vi "element_editor_hydrolysis_initial.vi"(9 "Env. Dir":refnum<vi>, 10 "Env. Ready?":refnum<vi>, 11 "Break":refnum<vi>) -> ()   [LabVIEW 2019]
uses:
  lib/libSimulationControl/libSimulationControl.lvlib
panel:
  # "*******************************************************************\nBiogas Plant Control\n\nAuthor: Paul Zügel\nGCSC-Frankfurt am Main 2020\n\n*******************************************************************"
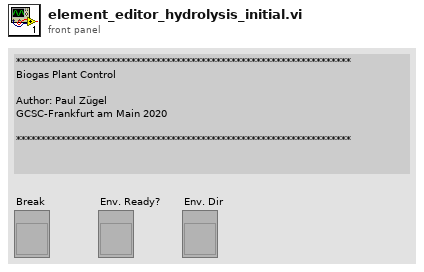
[diagram p1: front panel]
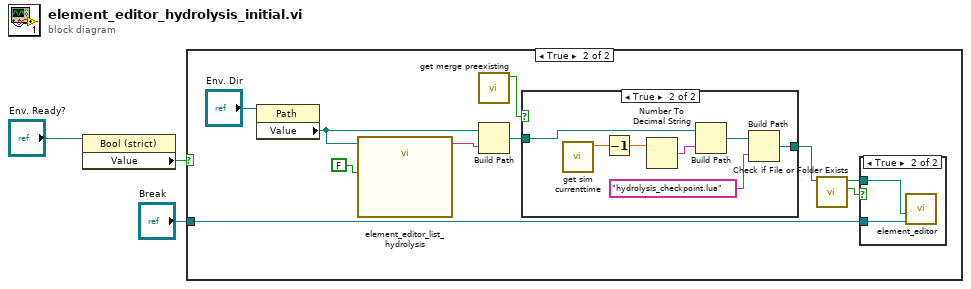
[diagram p0: block diagram]
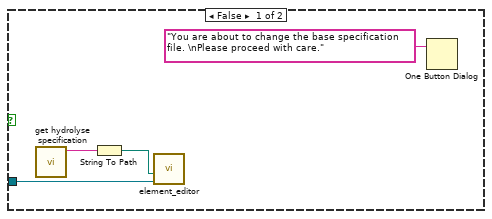
[diagram p2: hidden frame]
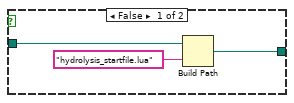
[diagram p3: hidden frame]
diagram:
  n1 = property class="Bool (strict)"(reference="Env. Ready?") -> ("Value"=w2:bool)  [unwired: 1 in, 2 out]
  n2 = case shown="True" w2 {
    tunnel: "Break" -> [w7 w13]
    frame False {
      n3 = call "get hydrolyse specification.vi"() -> ("function return"=w6:string)  [unwired: 10 in, 1 out]
      n4 = String To Path(string=w6) -> (path=w5:path)
      n5 = call "element_editor.vi"("Break"=w7, "LUA Specification File"=w5) -> ()  [unwired: 5 in, 1 out]
      n6 = One Button Dialog(message="You are about to change the base specification file. \nPlease proceed with care.") -> ()  [unwired: 1 in, 1 out]
    }
    frame True {
      n7 = property on="Property Node" class="Path"(reference="Env. Dir") -> ("Value"=w16:path)  [unwired: 1 in, 2 out]
      n8 = call "element_editor_list_hydrolysis.vi"("Allow all?"=FALSE, "path"=w16) -> ("Value"=w15:string)  [unwired: 6 in, 3 out]
      n9 = call "get merge preexisting.vi"() -> ("function return"=w10:bool)  [unwired: 10 in, 1 out]
      n10 = Build Path(base path=w16, name or relative path=w15) -> (appended path=w9:path)
      n11 = case shown="True" w10 {
        tunnel: w9 -> [w19 w27]
        tunnel: [w18 w23] -> w8
        frame False {
          n12 = Build Path(base path=w19, name or relative path="hydrolysis_startfile.lua") -> (appended path=w18:path)
        }
        frame True {
          n13 = call "get sim currenttime.vi"() -> ("current_time"=w22:dbl)  [unwired: 10 in, 1 out]
          n14 = Decrement(x=w22) -> (x-1=w21:dbl)
          n15 = Number To Decimal String(number=w21) -> (decimal integer string=w26:string)  [unwired: 1 in]
          n16 = Build Path(base path=w27, name or relative path=w26) -> (appended path=w25:path)
          n17 = Build Path(base path=w25, name or relative path="hydrolysis_checkpoint.lua") -> (appended path=w23:path)
        }
      }
      n18 = call <vilib>:"Check if File or Folder Exists.vi"("path"=w8) -> ("file or folder exists?"=w14:bool, "dup path"=w11:path)  [unwired: 8 in, 1 out]
      n19 = case shown="True" w14 {
        tunnel: w13 -> [_ w29]
        tunnel: w11 -> [_ w28]
        frame False {
        }
        frame True {
          n20 = call "element_editor.vi"("Break"=w29, "LUA Specification File"=w28) -> ()  [unwired: 5 in, 1 out]
        }
      }
    }
  }
